vi "Execute.vi"(0 "Template SoftMotion Drive Interface Plug-in Class in":refnum<class "Template SoftMotion Drive Interface Plug-in Class.lvclass">, 5 "Execute In":T2 {"Digital outputs" format="%x"}, 7 "Read Data In":u8[](array[numeric]) format="%x", 9 "Write Data In":u8[](array[numeric]) format="%x", 11 "error in (no error)":errorcluster) -> (4 "Template SoftMotion Drive Interface Plug-in Class out":refnum<class "Template SoftMotion Drive Interface Plug-in Class.lvclass">, 6 "Execute Out":T1, 8 "Read Data Out":u8[](array[numeric]) format="%x", 10 "Write Data Out":u8[](array[numeric]) format="%x", 15 "error out":errorcluster)   [LabVIEW 2014, in "Template SoftMotion Drive Interface Plug-in Class.lvclass"]
uses:
  Template SoftMotion Drive Interface Plug-in Class.lvclass
  <vilib>/Motion/plugins/PluginFramework/nismSDIFramework.ExecuteInput.ctl
  <vilib>/Motion/plugins/PluginFramework/nismSDIFramework.ExecuteOutput.ctl
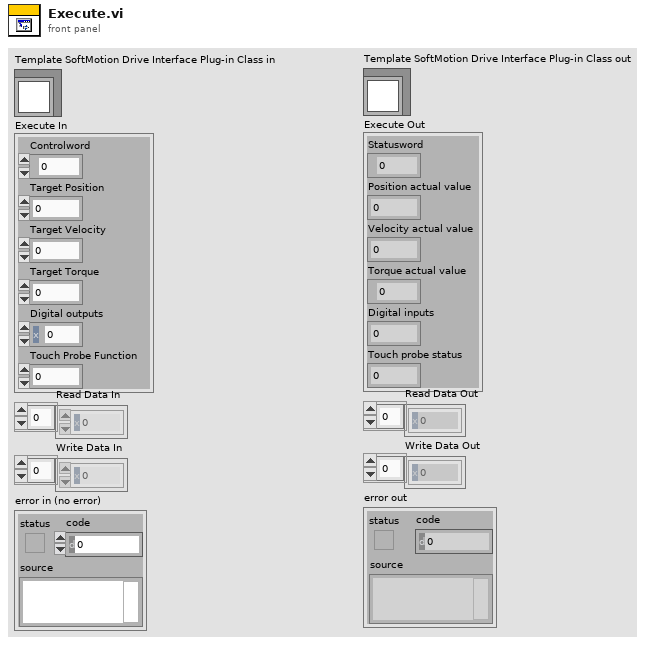
[diagram p1: front panel]
types:
  T1 = typedef "nismSDIFramework.ExecuteOutput.ctl" = cluster{"Statusword":u16, "Position actual value":i32, "Velocity actual value":i32, "Torque actual value":i16, "Digital inputs":u32, "Touch probe status":u16}
  T2 = typedef "nismSDIFramework.ExecuteInput.ctl" = cluster{"Controlword":u16, "Target Position":i32, "Target Velocity":i32, "Target Torque":i16, "Digital outputs":u32, "Touch Probe Function":u16}
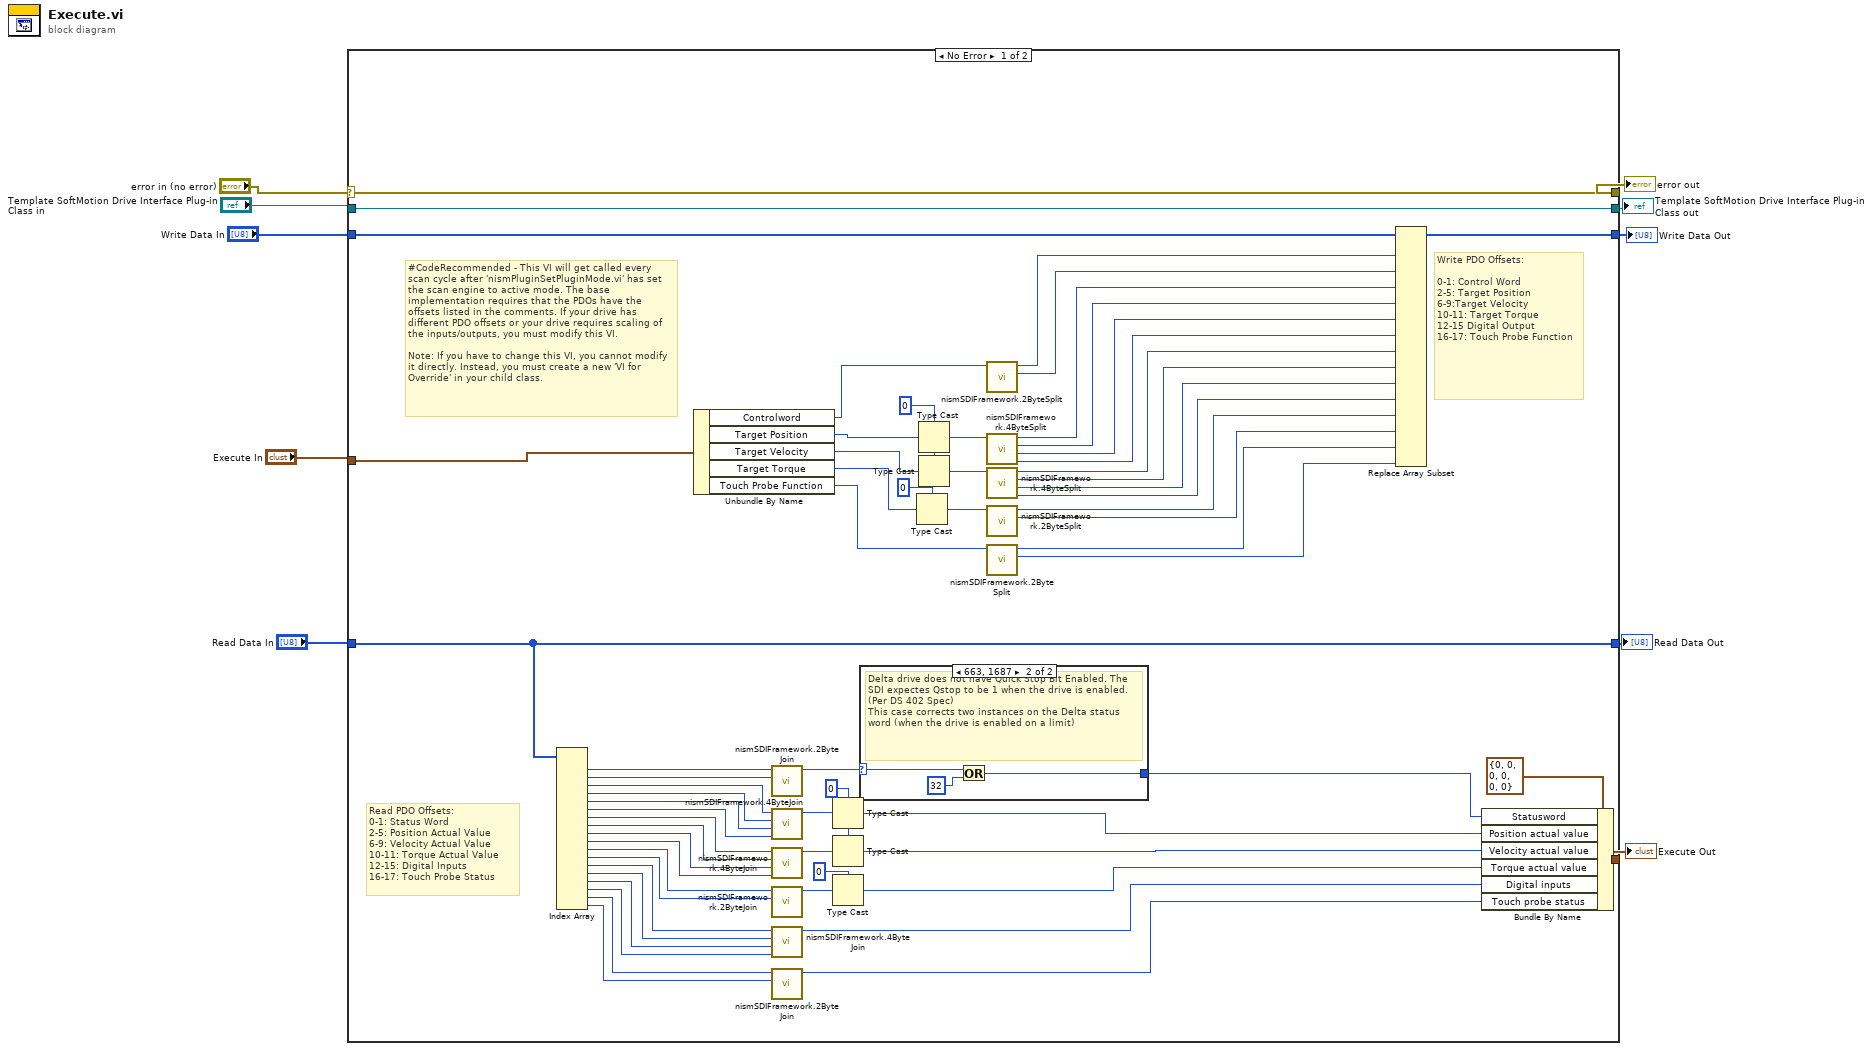
[diagram p0: block diagram]
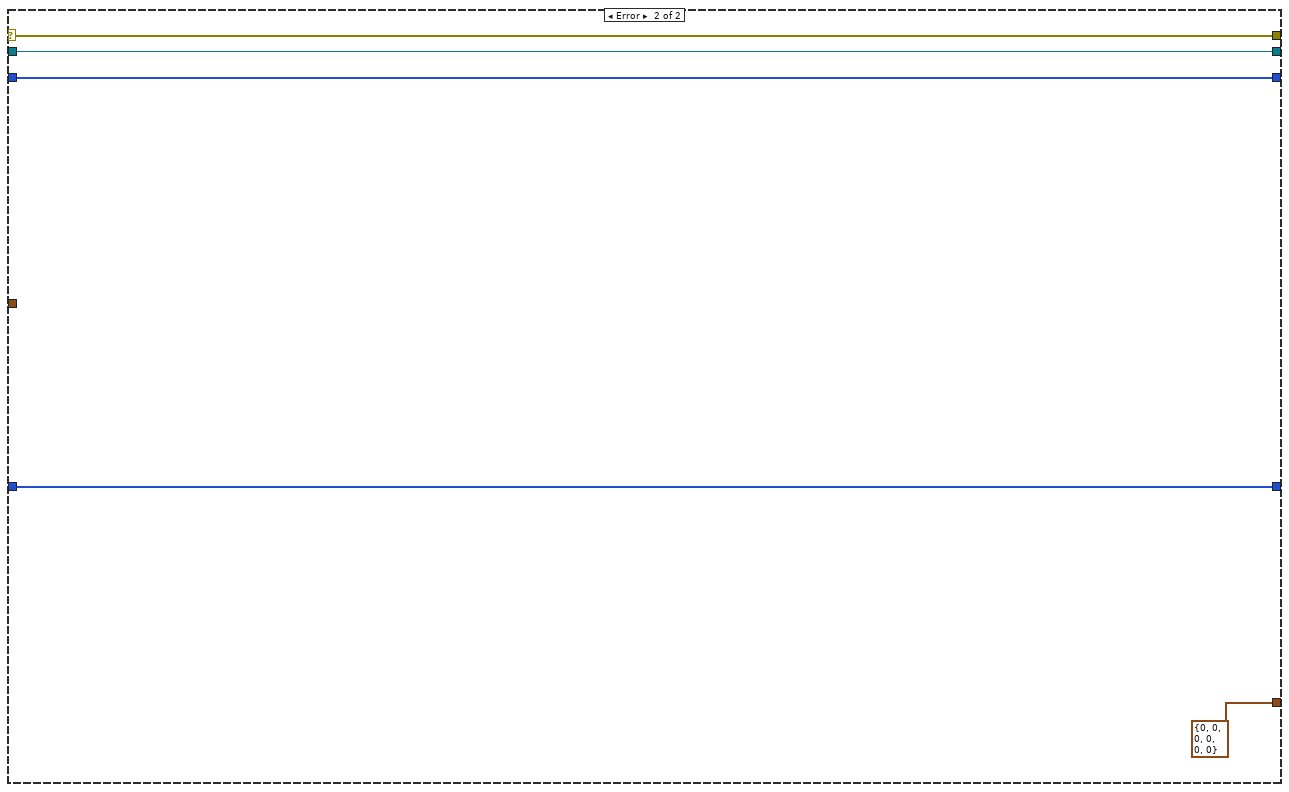
[diagram p3: hidden frame]
diagram:
  n1 = case shown="No Error" "error in (no error)" {
    selector: "error in (no error)" -> [w43 w81]
    tunnel: [w43 w81] -> w4
    tunnel: [w72 w80] -> w5
    tunnel: "Template SoftMotion Drive Interface Plug-in Class in" -> [w72 w80]
    tunnel: [w48 w79] -> w1
    tunnel: [w46 w77] -> w2
    tunnel: [w47 T1 {"Statusword"=0, "Position actual value"=0, "Velocity actual value"=0, "Torque actual value"=0, "Digital inputs"=0, "Touch probe status"=0} ("Execute Out")] -> w3
    tunnel: "Read Data In" -> [w46 w77]
    tunnel: "Execute In" -> [w45 _]
    tunnel: "Write Data In" -> [w44 w79]
    frame No Error {
      w49 = 0
      w40 = u32 0
      # "#CodeRecommended - This VI will get called every scan cycle after 'nismPluginSetPluginMode.vi' has set the scan engine to active mode. The base implementation requires that the PDOs have the offsets listed in the comments. If your drive has different PDO offsets or your drive requires scaling of the inputs/outputs, you must modify this VI.\n\nNote: If you have to change this VI, you cannot modify it directly. Instead, you must create a new 'VI for Override' in your child class."
      # "Read PDO Offsets:\n0-1: Status Word\n2-5: Position Actual Value\n6-9: Velocity Actual Value\n10-11: Torque Actual Value\n12-15: Digital Inputs\n16-17: Touch Probe Status"
      # "Write PDO Offsets: \n\n0-1: Control Word\n2-5: Target Position\n6-9:Target Velocity\n10-11: Target Torque\n12-15 Digital Output\n16-17: Touch Probe Function"
      n2 = Index Array(array=w46) -> (element #1=w69:u8, element #2=w68:u8, element #3=w56:u8, element #4=w55:u8, element #5=w54:u8, element #6=w53:u8, element #7=w60:u8, element #8=w59:u8, element #9=w58:u8, element #10=w57:u8, element #11=w28:u8, element #12=w27:u8, element #13=w22:u8, element #14=w21:u8, element #15=w20:u8, element #16=w19:u8, element #17=w18:u8, element #18=w17:u8)  [unwired: 18 in]
      n3 = Unbundle By Name(w45) -> ("Controlword"=w12:u16, "Target Position"=w71:i32, "Target Velocity"=w41:i32, "Target Torque"=w34:i16, "Touch Probe Function"=w29:u16)
      n4 = call <vilib>:"nismSDIFramework.2ByteJoin.vi"("hi"=w68, "lo"=w69) -> ("2 bytet out"=w13:u16)  [unwired: 9 in]
      n5 = call <vilib>:"nismSDIFramework.4ByteJoin.vi"("hihi"=w53, "hilo"=w54, "lohi"=w55, "lolo"=w56) -> ("4 byte out"=w52:u32)  [unwired: 7 in]
      n6 = call <vilib>:"nismSDIFramework.4ByteJoin.vi"("hihi"=w57, "hilo"=w58, "lohi"=w59, "lolo"=w60) -> ("4 byte out"=w50:u32)  [unwired: 7 in]
      n7 = call <vilib>:"nismSDIFramework.2ByteJoin.vi"("hi"=w27, "lo"=w28) -> ("2 bytet out"=w26:u16)  [unwired: 9 in]
      n8 = call <vilib>:"nismSDIFramework.4ByteJoin.vi"("hihi"=w19, "hilo"=w20, "lohi"=w21, "lolo"=w22) -> ("4 byte out"=w23:u32)  [unwired: 7 in]
      n9 = call <vilib>:"nismSDIFramework.2ByteJoin.vi"("hi"=w17, "lo"=w18) -> ("2 bytet out"=w16:u16)  [unwired: 9 in]
      n10 = Type Cast(type=w49, x=w52) -> (*(type *) &x=w51:i32)
      n11 = Type Cast(type=w49, x=w50) -> (*(type *) &x=w42:i32)
      n12 = Type Cast(type=i16 0, x=w26) -> (*(type *) &x=w24:i16)
      n13 = case shown="663, 1687" w13 {
        selector: w13 -> [w73 w76]
        tunnel: [w73 w74] -> w11
        frame 0, Default {
        }
        frame 663, 1687 {
          # "Delta drive does not have Quick Stop Bit Enabled. The SDI expectes Qstop to be 1 when the drive is enabled. (Per DS 402 Spec)\nThis case corrects two instances on the Delta status word (when the drive is enabled on a limit)"
          n14 = Or(x=w76, y=u16 32) -> (x .or. y?=w74:u16)
        }
      }
      n15 = Type Cast(type=u16 0, x=w34) -> (*(type *) &x=w32:u16)
      n16 = Type Cast(type=w40, x=w71) -> (*(type *) &x=w61:u32)
      n17 = Type Cast(type=w40, x=w41) -> (*(type *) &x=w35:u32)
      n18 = call <vilib>:"nismSDIFramework.2ByteSplit.vi"("2 byte in"=w12) -> ("hi"=w66:u8, "lo"=w67:u8)  [unwired: 9 in]
      n19 = call <vilib>:"nismSDIFramework.4ByteSplit.vi"("4 byte in"=w61) -> ("hihi"=w62:u8, "hilo"=w63:u8, "lohi"=w64:u8, "lolo"=w65:u8)  [unwired: 7 in]
      n20 = call <vilib>:"nismSDIFramework.4ByteSplit.vi"("4 byte in"=w35) -> ("hihi"=w36:u8, "hilo"=w37:u8, "lohi"=w38:u8, "lolo"=w39:u8)  [unwired: 7 in]
      n21 = call <vilib>:"nismSDIFramework.2ByteSplit.vi"("2 byte in"=w32) -> ("hi"=w30:u8, "lo"=w31:u8)  [unwired: 9 in]
      n22 = call <vilib>:"nismSDIFramework.2ByteSplit.vi"("2 byte in"=w29) -> ("hi"=w14:u8, "lo"=w15:u8)  [unwired: 9 in]
      n23 = Replace Array Subset(array=w44, new element #1=w67, new element #2=w66, new element #3=w65, new element #4=w64, new element #5=w63, new element #6=w62, new element #7=w39, new element #8=w38, new element #9=w37, new element #10=w36, new element #11=w31, new element #12=w30, new element #13=w15, new element #14=w14) -> (w48:u8[])  [unwired: 14 in]
      n24 = Bundle By Name(cluster=T1 {"Statusword"=0, "Position actual value"=0, "Velocity actual value"=0, "Torque actual value"=0, "Digital inputs"=0, "Touch probe status"=0} ("Execute Out"), "Statusword"=w11, "Position actual value"=w51, "Velocity actual value"=w42, "Torque actual value"=w24, "Digital inputs"=w23, "Touch probe status"=w16) -> (w47:T1)
    }
    frame Error {
    }
  }
  "error out" <- w4
  "Template SoftMotion Drive Interface Plug-in Class out" <- w5
  "Write Data Out" <- w1
  "Read Data Out" <- w2
  "Execute Out" <- w3
